vi "CheckSettingsNI-DAQ_Class.vi"(6 "Default value":T1={"Range"=10.0, "Input terminal configuration"=10106} {"Input terminal configuration" items=["default"=-1, "RSE"=10083, "NRSE"=10078, "Differential"=10106, "Pseudodifferential"=12529]}, 8 "error in (no error)":errorcluster, 9 "Ranges and couplings":T2 {"Input terminal configuration" items=["default"=-1, "RSE"=10083, "NRSE"=10078, "Differential"=10106, "Pseudodifferential"=12529]}, 10 "Physical channels":string[](array[string]), 11 "Number of channels":i32) -> (0 "error out":errorcluster, 1 "Ranges and couplings  out":T2 {"Input terminal configuration" items=["default"=-1, "RSE"=10083, "NRSE"=10078, "Differential"=10106, "Pseudodifferential"=12529]}, 2 "Physical channels out":string[](array[string]))   [LabVIEW 2015]
uses:
  Controls/Ranges and coupling.ctl
  Controls/Range and coupling.ctl
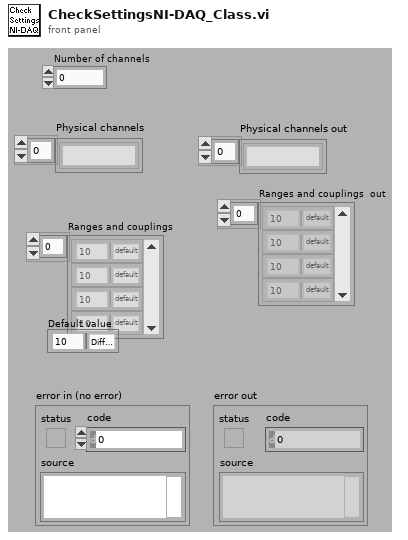
[diagram p1: front panel]
types:
  T1 = typedef "Range and coupling.ctl" = cluster{"Range":dbl, "Input terminal configuration":i32}
  T2 = typedef "Ranges and coupling.ctl" = T1[]
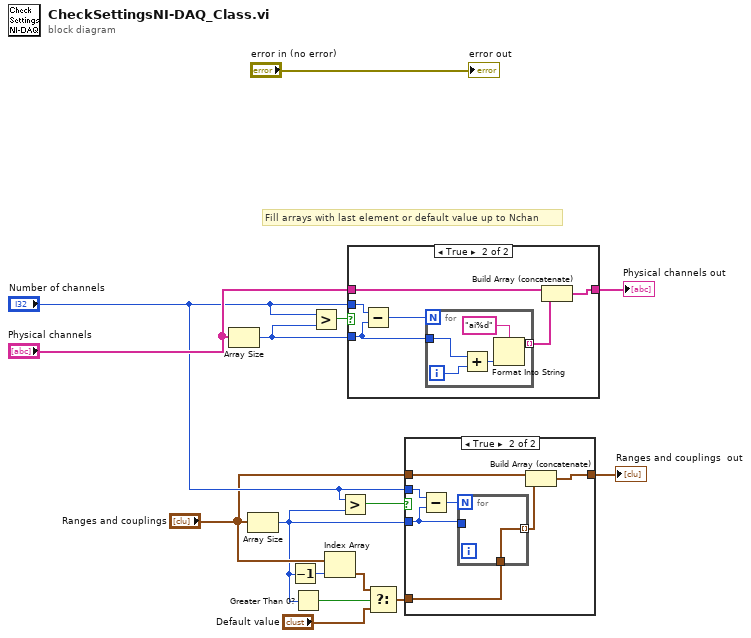
[diagram p0: block diagram]
diagram:
  # "Fill arrays with last element or default value up to Nchan"
  n1 = Array Size(array="Physical channels") -> (size(s)=w14:i32)
  n2 = Array Size(array="Ranges and couplings") -> (size(s)=w6:i32)
  n3 = Decrement(x=w6) -> (x-1=w7:i32)
  n4 = Greater Than 0?(x=w6) -> (x > 0?=w5:bool)
  n5 = Greater?(x="Number of channels", y=w14) -> (0:w15:bool)
  n6 = Index Array(array="Ranges and couplings", index=w7) -> (element=w4:T1)
  n7 = Greater?(x="Number of channels", y=w6) -> (0:w10:bool)
  n8 = case shown="True" w15 {
    tunnel: "Number of channels" -> [_ w22]
    tunnel: w14 -> [_ w19]
    tunnel: "Physical channels" -> [w16 w20]
    tunnel: [w16 w17] -> w11
    frame False {
    }
    frame True {
      n9 = Subtract(x=w22, y=w19) -> (x-y=w18:i32)
      n10 = for {
        N: w18 -> [_]
        tunnel: [w23] -> w21 mode=indexing
        tunnel: w19 -> [w26]
        i -> [w27]
        n11 = Add(x=w26, y=w27) -> (x+y=w24:i32)
        n12 = Format Into String(format string="ai%d", w24) -> (resulting string=w23:string)  [unwired: 2 in, 1 out]
      }
      n13 = Build Array (concatenate)(w20, w21) -> (w17:string[])
    }
  }
  "Physical channels out" <- w11
  n14 = Select(t=w4, s=w5, f="Default value") -> (s? t:f=w3:T1)
  n15 = case shown="True" w10 {
    tunnel: "Number of channels" -> [_ w35]
    tunnel: w6 -> [_ w32]
    tunnel: "Ranges and couplings" -> [w28 w33]
    tunnel: [w28 w30] -> w2
    tunnel: w3 -> [_ w29]
    frame False {
    }
    frame True {
      n16 = Subtract(x=w35, y=w32) -> (x-y=w31:i32)
      n17 = for {
        N: w31 -> [_]
        tunnel: [w36] -> w34 mode=indexing
        tunnel: w32 -> [_]
        tunnel: w29 -> [w36]
      }
      n18 = Build Array (concatenate)(w33, w34) -> (w30:T2)
    }
  }
  "Ranges and couplings  out" <- w2
  "error out" <- "error in (no error)"
